vi "Init OOB.vi"(8 "error in (no error)":errorcluster, 10 "Cases to Skip Payload":u8[](array[numeric]), 11 "OOB in":refnum<class "CIFOutOfBand.lvclass">) -> (0 "error out":errorcluster, 3 "OOB out":refnum<class "CIFOutOfBand.lvclass">)   [LabVIEW 2021, in "CIFOutOfBand.lvclass"]
doc: "This will initialize the communication mechanism (DVR with bitwise command register and variant for payload data) between the time critical loop and the out of band communication loop. \n\nEach OOB mechanism will support up to 64 unique commands. \nTo support multi-rate operations multiple commands can be held in the DVR. \nManagement of the payload should be handled by higher level code calling this library. If multiple commands with payload are possible best practice is the payload consists of a cluster with multiple data elements. \n\nCases to Skip Payload is an array of the commands that will not contain payloads. These commands will be passed but no payload data will be transfered. This is optional but will improve performance for commands with no payload."
uses:
  CIFOutOfBand.lvclass
  Typedef/OOB Container.ctl
  CIFOutOfBand.lvclass/CIFOutOfBand.ctl
  Accessors/Write Payload Mask.vi
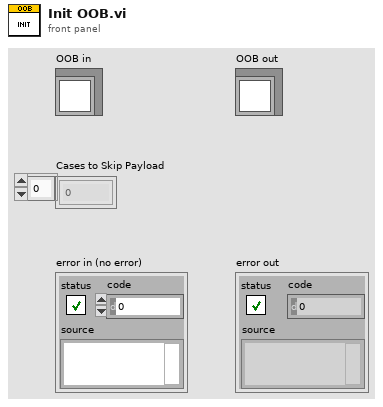
[diagram p1: front panel]
types:
  T1 = typedef "CIFOutOfBand.lvclass/OOB Container.ctl" = cluster{"Commands":u64, "Payload":variant}
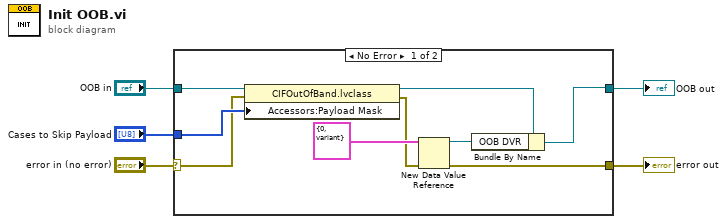
[diagram p0: block diagram]
diagram:
  n1 = case shown="No Error" "error in (no error)" {
    selector: "error in (no error)" -> [w7 w16]
    tunnel: [w6 w16] -> w4
    tunnel: [w9 w15] -> w3
    tunnel: "OOB in" -> [w11 w15]
    tunnel: "Cases to Skip Payload" -> [w12 _]
    frame No Error {
      n2 = property class="CIFOutOfBand.lvclass"(reference=w11, error in=w7, "Accessors:Payload Mask"=w12) -> (reference out=w10:refnum<class "CIFOutOfBand.lvclass">, error out=w8:errorcluster)
      n3 = New Data Value Reference(data value=T1 {"Commands"=0, "Payload"=variant} ("OOB Container"), error in=w8) -> (data value reference=w13:refnum<data-value>, error out=w6:errorcluster)
      n4 = Bundle By Name(cluster=w10, "OOB DVR"=w13) -> (w9:refnum<class "CIFOutOfBand.lvclass">)
    }
    frame Error {
    }
  }
  "error out" <- w4
  "OOB out" <- w3
